vi "2.vi"() -> ()   [LabVIEW 2020]
uses:
  <vilib>/numeric/Random Number (Range) U64.vi
panel:
  out "XY Graph 2":cluster{"Y":dbl[], "Y":dbl[]}[](graph)
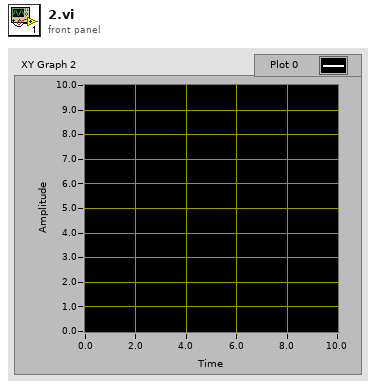
[diagram p1: front panel]
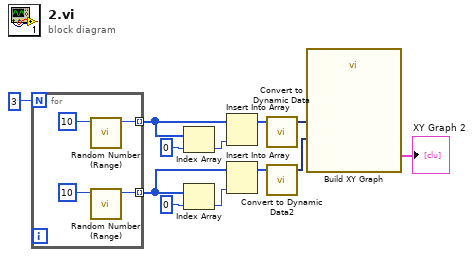
[diagram p0: block diagram]
diagram:
  n1 = for {
    N: 3 -> [_]
    tunnel: [w14] -> w7 mode=indexing
    tunnel: [w13] -> w1 mode=indexing
    n2 = call-poly <vilib>:"Random Number (Range).vi"("upper bound (100)"=u64 10) -> ("number"=w14:u64)  [unwired: 10 in]
    n3 = call-poly <vilib>:"Random Number (Range).vi"("upper bound (100)"=u64 10) -> ("number"=w13:u64)  [unwired: 10 in]
  }
  n4 = Index Array(array=w7, index=0) -> (element=w6:u64)
  n5 = Index Array(array=w1, index=0) -> (element=w5:u64)
  n6 = Insert Into Array(array=w7, new element=w6) -> (w2:u64[])  [unwired: 1 in]
  n7 = Insert Into Array(array=w1, new element=w5) -> (w3:u64[])  [unwired: 1 in]
  n8 = call "Convert to Dynamic Data"("Array"=w2) -> ("Dynamic Data Type"=w10:dynamicdata)  [unwired: 3 in]
  n9 = call "Convert to Dynamic Data2"("Array"=w3) -> ("Dynamic Data Type"=w9:dynamicdata)  [unwired: 3 in]
  n10 = call "Build XY Graph"("Y Input"=w9, "X Input"=w10) -> ("XY Graph"=→"XY Graph 2":cluster{"X":dbl[], "Y":dbl[]}[])  [unwired: 8 in, 1 out]
